vi "Measure.vi"(8 "error in":errorcluster, 9 "timeout":dbl=10.0 format="%0.2f", 10 "number of samples per channel":i32=-1, 11 "task/channels in":refnum<k21>) -> (0 "error out":errorcluster, 2 "data":dbl[][](array[numeric]) format="%0.2f", 3 "task out":refnum<k21>)   [LabVIEW 2023, in "AI.lvlib"]
uses:
  AI.lvlib
  <vilib>/DAQmx/read.llb/DAQmx Read (Analog 2D DBL NChan NSamp).vi
  <vilib>/DAQmx/miscellaneous.llb/DAQmx Fill In Error Info.vi
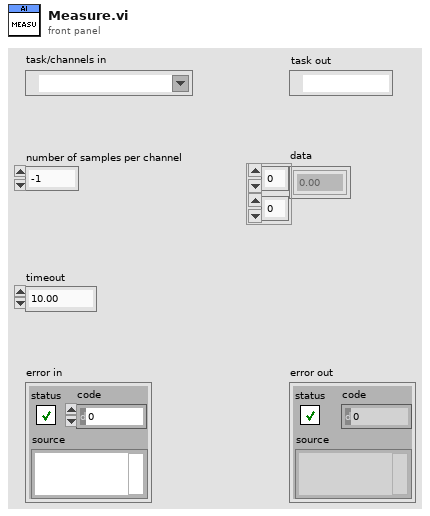
[diagram p1: front panel]
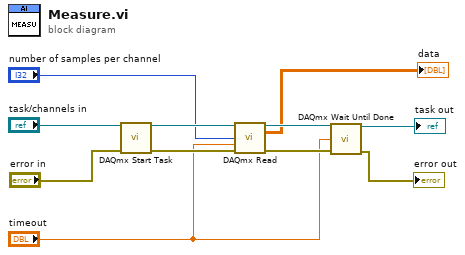
[diagram p0: block diagram]
diagram:
  n1 = call <vilib>:"DAQmx Start Task.vi"("task/channels in"="task/channels in", "error in"="error in") -> ("task out"=w9:refnum<k21>, "error out"=w8:errorcluster)  [unwired: 12 in]
  n2 = call-poly <vilib>:"DAQmx Read.vi"("task/channels in"=w9, "number of samples per channel"="number of samples per channel", "timeout"="timeout", "error in"=w8) -> ("task out"=w6:refnum<k21>, "data"=→"data":dbl[][], "error out"=w5:errorcluster)  [unwired: 9 in]
  n3 = call <vilib>:"DAQmx Wait Until Done.vi"("task/channels in"=w6, "timeout (sec)"="timeout", "error in"=w5) -> ("task out"=→"task out":refnum<k21>, "error out"=→"error out":errorcluster)  [unwired: 11 in]
